vi "permute_sensor_lut.vi"(11 "Sensor LUT in":sgl[][][](array[numeric]) format="%#_3p") -> (3 "Sensor LUT out":sgl[][][](array[numeric]) format="%#_3p")   [LabVIEW 2013]
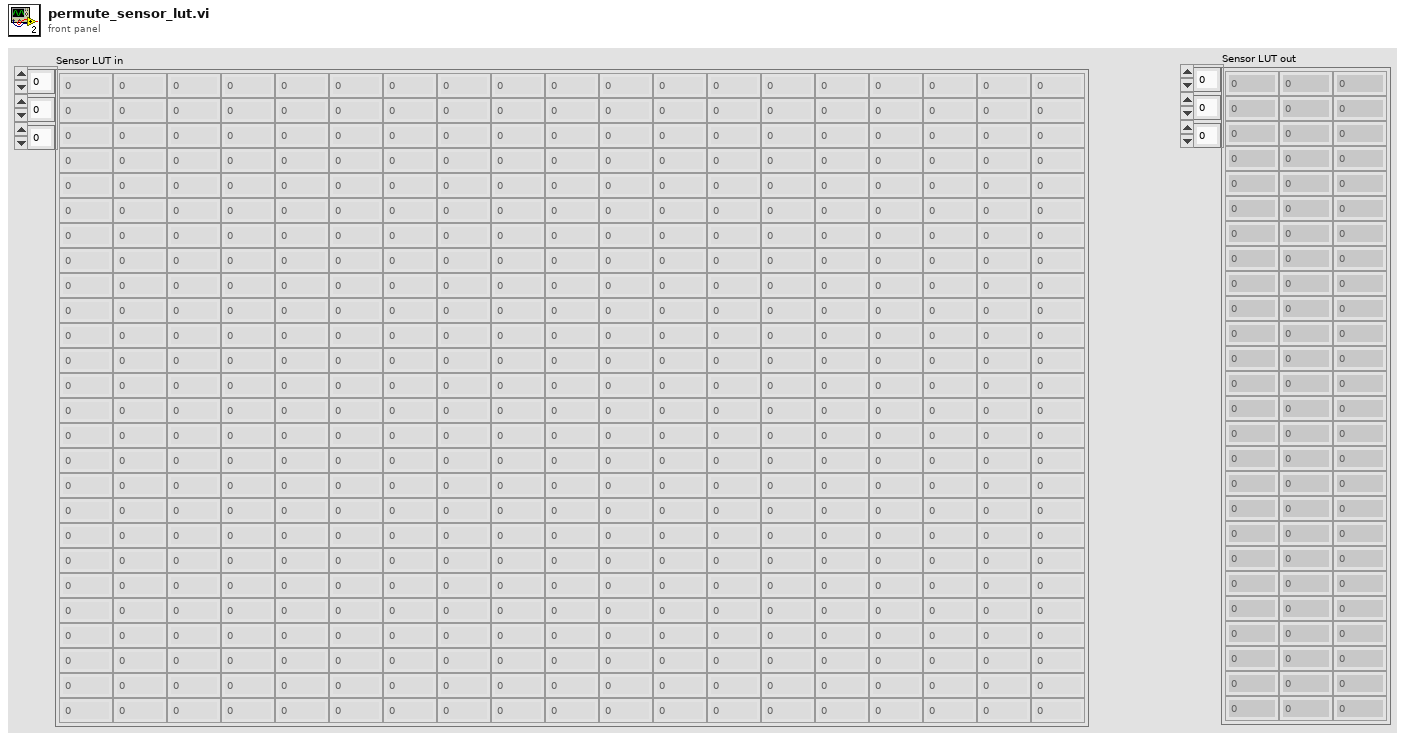
[diagram p1: front panel]
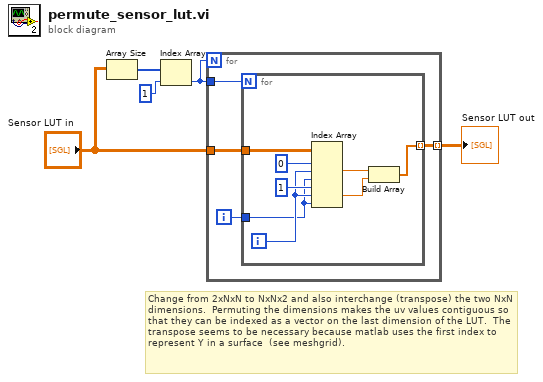
[diagram p0: block diagram]
diagram:
  # "Change from 2xNxN to NxNx2 and also interchange (transpose) the two NxN dimensions.  Permuting the dimensions makes the uv values contiguous so that they can be indexed as a vector on the last dimension of the LUT.  The transpose seems to be necessary because matlab uses the first index to represent Y in a surface  (see meshgrid)."
  n1 = Array Size(array="Sensor LUT in") -> (size(s)=w2:i32[])
  n2 = Index Array(array=w2, index=1) -> (element=w3:i32)
  n3 = for {
    N: w3 -> [_]
    tunnel: w3 -> [w9]
    tunnel: "Sensor LUT in" -> [w8]
    tunnel: [w6] -> w4 mode=indexing
    i -> [w7]
    n4 = for {
      N: w9 -> [_]
      tunnel: w8 -> [w17]
      tunnel: w7 -> [w10]
      tunnel: [w12] -> w6 mode=indexing
      i -> [w11]
      n5 = Index Array(array=w17, index (dim 0) #1=0 ("disabled index (page)"), index (dim 1) #1=w11, index (dim 2) #1=w10, index (dim 0) #2=1 ("index (page)"), index (dim 1) #2=w11, index (dim 2) #2=w10) -> (element #1=w15:sgl, element #2=w14:sgl)
      n6 = Build Array(w15, w14) -> (w12:sgl[])
    }
  }
  "Sensor LUT out" <- w4
